vi "vimUpdate.vi"() -> ()   [LabVIEW 2014, in "lv-cli-steps.lvlib"]
uses:
  lv-cli-steps.lvlib
  <vilib>/Utility/error.llb/DialogType.ctl
  <vilib>/Wiresmith Technology/LabVIEW CLI/CLI Class/CLI.lvclass
  <vilib>/JKI/VIPM API/VIPM API_vipm_api.lvlib
panel:
  out "error out":errorcluster
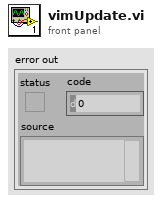
[diagram p1: front panel]
types:
  T1 = typedef "DialogType.ctl" = u16
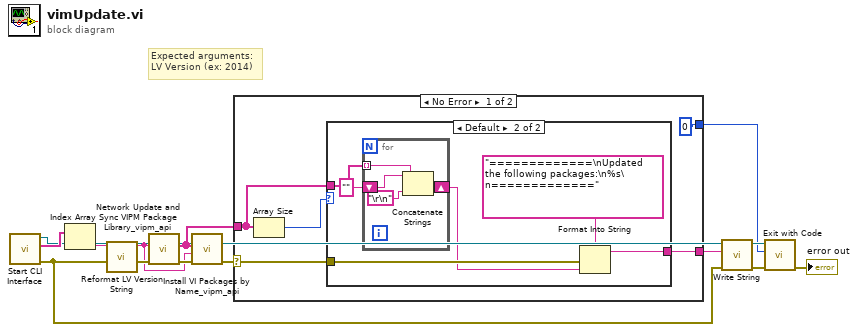
[diagram p0: block diagram]
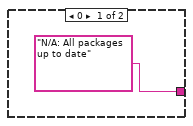
[diagram p2: hidden frame]
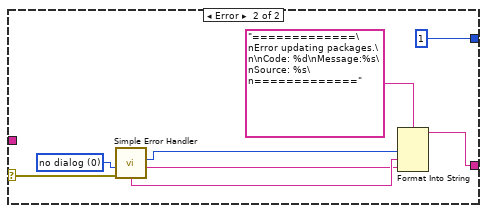
[diagram p3: hidden frame]
diagram:
  # "Expected arguments:\nLV Version (ex: 2014)"
  n1 = call <vilib>:"Start CLI Interface.vi"() -> ("error out"=w4:errorcluster, "Custom Parameters"=w13:string[], "CLI out"=w11:refnum<class "CLI.lvclass">)  [unwired: 9 in]
  n2 = Index Array(array=w13) -> (element=w3:string)  [unwired: 1 in]
  n3 = call "Reformat LV Version String.vi"("Version String (2014)"=w3) -> ("Short Version String (14.0)"=w1:string)  [unwired: 10 in]
  n4 = call <vilib>:"Network Update and Sync VIPM Package Library_vipm_api.vi"("error in (no error)"=w4, "LabVIEW Version"=w1) -> ("error out"=w6:errorcluster, "New Package Updates"=w2:string[])  [unwired: 8 in]
  n5 = call <vilib>:"Install VI Packages by Name_vipm_api.vi"("error in (no error)"=w6, "LabVIEW Version"=w1, "Package Names to Install []"=w2) -> ("error out"=w5:errorcluster)  [unwired: 8 in]
  n6 = case shown="No Error" w5 {
    selector: w5 -> [w18 w36]
    tunnel: w2 -> [w14 _]
    tunnel: [w17 w37] -> w12
    tunnel: [0 ("Exit Code (0)") 1 ("Exit Code (0)")] -> w8
    frame No Error {
      n7 = Array Size(array=w14) -> (size(s)=w15:i32)
      n8 = case shown="Default" w15 {
        tunnel: w18 -> [_ w24]
        tunnel: ["N/A: All packages up to date" w23] -> w17
        tunnel: w14 -> [_ w22]
        frame 0 {
        }
        frame Default {
          n9 = for {
            tunnel: w22 -> [w29] mode=indexing
            shift-right: [w27] -> w20
            shift-left: "" -> [w26]
            n10 = Concatenate Strings(w26, w29, "\r\n") -> (w27:string)
          }
          n11 = Format Into String(format string="=============\nUpdated the following packages:\n%s\n=============", error in=w24, w20) -> (resulting string=w23:string)  [unwired: 1 in, 1 out]
        }
      }
    }
    frame Error {
      w35 = T1 0 items=["no dialog", "OK message", "continue or stop message", "OK message + warnings", "continue/stop + warnings"] ("type of dialog (OK msg:1)")
      n12 = call <vilib>:"Simple Error Handler.vi"("type of dialog (OK msg:1)"=w35, "error in (no error)"=w36) -> ("code out"=w32:i32, "source out"=w30:string, "message"=w31:string)  [unwired: 3 in, 2 out]
      n13 = Format Into String(format string="=============\nError updating packages.\n\nCode: %d\nMessage:%s\nSource: %s\n=============", w32, w31, w30) -> (resulting string=w37:string)  [unwired: 2 in, 1 out]
    }
  }
  n14 = call <vilib>:"Write String.vi"("error in (no error)"=w4, "Text to Write"=w12, "CLI in"=w11) -> ("error out"=w10:errorcluster, "CLI out"=w9:refnum<class "CLI.lvclass">)  [unwired: 7 in]
  n15 = call <vilib>:"Exit with Code.vi"("error in (no error)"=w10, "Exit Code (0)"=w8, "CLI in"=w9) -> ("error out"=→"error out":errorcluster)  [unwired: 8 in]
